vi "RANGE Update Meter Types.vi"(0 "Start Up File in":string[][](array[string]), 1 "Meter Type 1":string, 2 "Meter Type 2":string, 3 "Meter Type 3":string, 4 "Meter Type 4":string, 5 "Error In":errorcluster, 7 "Meter Type 5":string, 9 "Meter Type 6":string) -> (14 "Start Up File out":string[][](array[string]), 19 "Error Out":errorcluster)   [LabVIEW 2023]
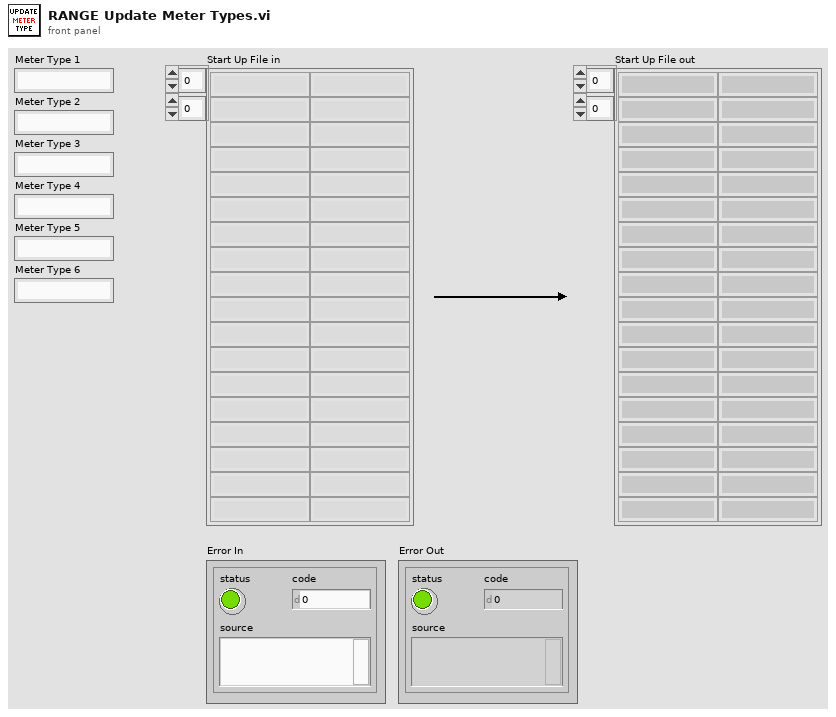
[diagram p1: front panel]
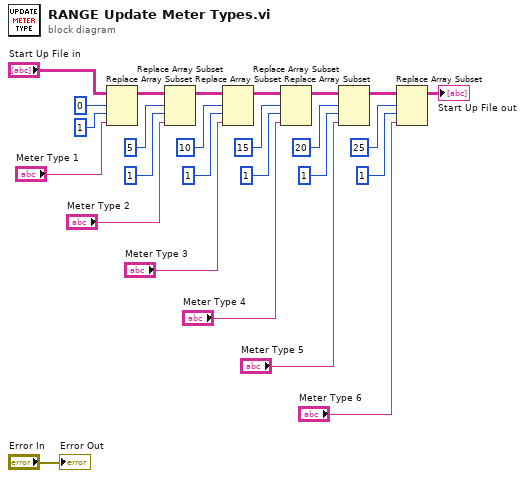
[diagram p0: block diagram]
diagram:
  n1 = Replace Array Subset(array="Start Up File in", new element="Meter Type 1", index (row)=0 ("disabled index (row)"), index (col)=1 ("disabled index (col)")) -> (w21:string[][])
  n2 = Replace Array Subset(array=w21, new element="Meter Type 2", index (row)=5 ("disabled index (row)"), index (col)=1 ("disabled index (col)")) -> (w22:string[][])
  n3 = Replace Array Subset(array=w22, new element="Meter Type 3", index (row)=10 ("disabled index (row)"), index (col)=1 ("disabled index (col)")) -> (w23:string[][])
  n4 = Replace Array Subset(array=w23, new element="Meter Type 4", index (row)=15 ("disabled index (row)"), index (col)=1 ("disabled index (col)")) -> (w24:string[][])
  n5 = Replace Array Subset(array=w24, new element="Meter Type 5", index (row)=20 ("disabled index (row)"), index (col)=1 ("disabled index (col)")) -> (w25:string[][])
  n6 = Replace Array Subset(array=w25, new element="Meter Type 6", index (row)=25 ("disabled index (row)"), index (col)=1 ("disabled index (col)")) -> (→"Start Up File out":string[][])
  "Error Out" <- "Error In"
